vi "Query Capabilities (Trip).vi"(0 "VISA resource name":refnum<visa-resource-name>, 5 "Absolute Maximums (T)":bool=TRUE, 11 "error in (no error)":errorcluster) -> (4 "VISA resource name out":refnum<visa-resource-name>, 6 "Minimum (s)":dbl, 8 "Maximum (s)":dbl, 15 "error out":errorcluster)   [LabVIEW 2012, in "NH Research Regenerative Test Series.lvlib"]
doc: "This will query the absolute minimum and maximum trip time setting for the Module."
uses:
  <instrlib>/NH Research Regenerative Test Series/NH Research Regenerative Test Series.lvlib
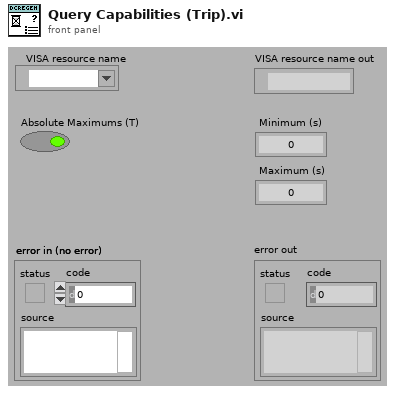
[diagram p1: front panel]
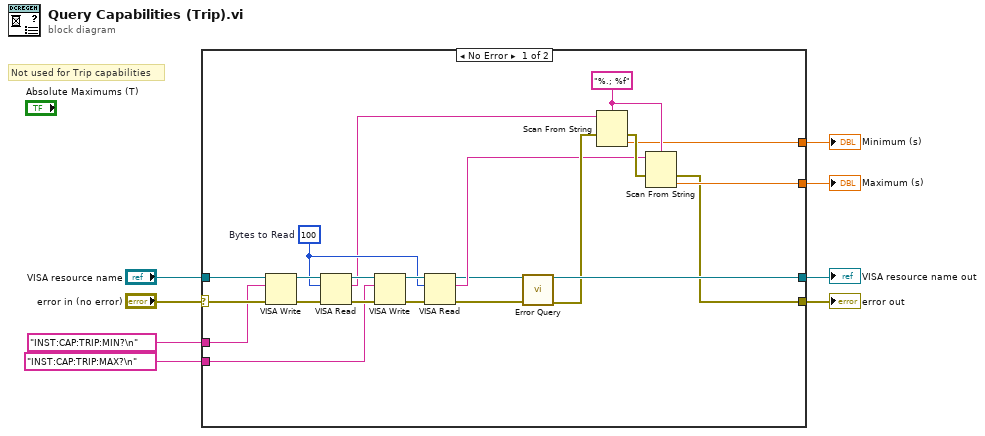
[diagram p0: block diagram]
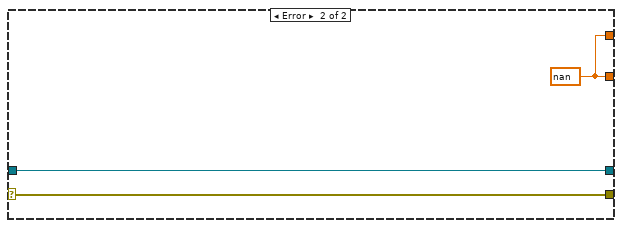
[diagram p2: hidden frame]
diagram:
  # "Not used for Trip capabilities"
  n1 = case shown="No Error" "error in (no error)" {
    selector: "error in (no error)" -> [w28 w33]
    tunnel: [w9 w33] -> w7
    tunnel: [w26 w32] -> w5
    tunnel: "VISA resource name" -> [w27 w32]
    tunnel: "INST:CAP:TRIP:MIN?\n" ("write buffer") -> [w21 _]
    tunnel: "INST:CAP:TRIP:MAX?\n" ("write buffer") -> [w20 _]
    tunnel: [w16 w31] -> w1
    tunnel: [w12 w31] -> w2
    frame No Error {
      w13 = "%.; %f" ("format string")
      w18 = u32 100  # Bytes to Read
      n2 = VISA Write(VISA resource name=w27, write buffer=w21, error in (no error)=w28) -> (VISA resource name out=w29:refnum<visa-resource-name>, error out=w30:errorcluster)  [unwired: 1 out]
      n3 = VISA Read(VISA resource name=w29, byte count=w18, error in (no error)=w30) -> (VISA resource name out=w19:refnum<visa-resource-name>, read buffer=w15:string, error out=w22:errorcluster)  [unwired: 1 out]
      n4 = VISA Write(VISA resource name=w19, write buffer=w20, error in (no error)=w22) -> (VISA resource name out=w23:refnum<visa-resource-name>, error out=w24:errorcluster)  [unwired: 1 out]
      n5 = VISA Read(VISA resource name=w23, byte count=w18, error in (no error)=w24) -> (VISA resource name out=w10:refnum<visa-resource-name>, read buffer=w14:string, error out=w11:errorcluster)  [unwired: 1 out]
      n6 = call <instrlib>:"Error Query.vi"("VISA resource name"=w10, "error in (no error)"=w11) -> ("VISA resource name out"=w26:refnum<visa-resource-name>, "error out"=w25:errorcluster)  [unwired: 10 in, 2 out]
      n7 = Scan From String(format string=w13, input string=w15, error in=w25) -> (error out=w17:errorcluster, output 1=w12:dbl)  [unwired: 2 in, 2 out]
      n8 = Scan From String(format string=w13, input string=w14, error in=w17) -> (error out=w9:errorcluster, output 1=w16:dbl)  [unwired: 2 in, 2 out]
    }
    frame Error {
      w31 = nan
    }
  }
  "error out" <- w7
  "VISA resource name out" <- w5
  "Minimum (s)" <- w2
  "Maximum (s)" <- w1
